vi "PI.vi"(9 "u(k-1)_in":fxp<+,20,0>, 10 "e(k-1)_in":fxp<+/-,29,9>, 11 "e(k)_in":fxp<+/-,29,9>) -> (3 "u(k)_in":fxp<+,20,0>)   [LabVIEW 2015]
uses:
  <vilib>/rvi/FXPMathLib/FxpMul/XNode/nifxpmath_Multiplier.xnode
  <vilib>/rvi/FXPMathLib/FxpAdd/XNode/nifxpmath_Add.xnode
  <vilib>/rvi/FXPMathLib/sim/FxpSim.dll
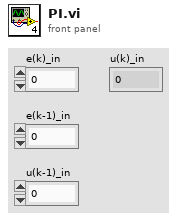
[diagram p1: front panel]
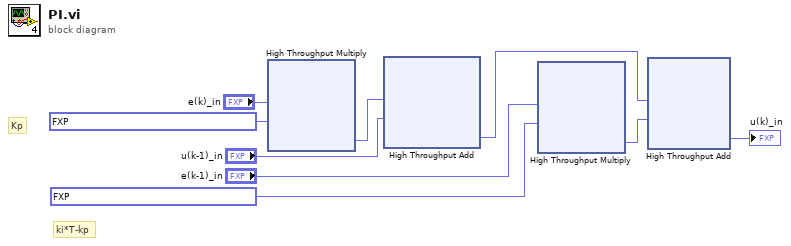
[diagram p0: block diagram]
diagram:
  # "Kp"
  # "ki*T-kp"
  n1 = xnode ("High Throughput Multiply")("x"="e(k)_in", "y"=fxp<+,32,0> 0.003999999957159162) -> ("x*y"=w4:fxp<+/-,61,9>)
  n2 = xnode ("High Throughput Add")("x"=w4, "y"="u(k-1)_in") -> ("x+y"=w2:fxp<+/-,62,10>)
  n3 = xnode ("High Throughput Multiply")("x"="e(k-1)_in", "y"=fxp<+/-,32,0> -0.003971999976783991) -> ("x*y"=w1:fxp<+/-,61,9>)
  n4 = xnode ("High Throughput Add")("x"=w2, "y"=w1) -> ("x+y"=→"u(k)_in":fxp<+,20,0>)
